vi "Get Connection Count.vi"(8 "error in (no error)":errorcluster, 11 "TCP Socket Server in":refnum<data-value>) -> (0 "error out":errorcluster, 2 "connection count":i32, 3 "TCP Socket Server out":refnum<data-value>)   [LabVIEW 2019, in "TCP Socket Server.lvclass"]
uses:
  TCP Socket Server.lvclass
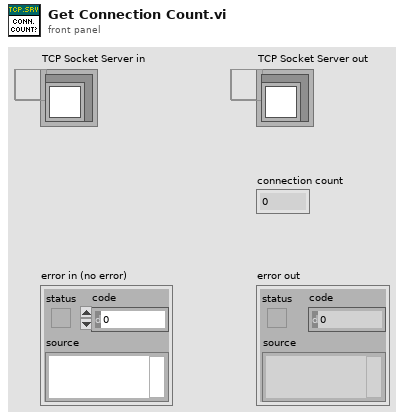
[diagram p1: front panel]
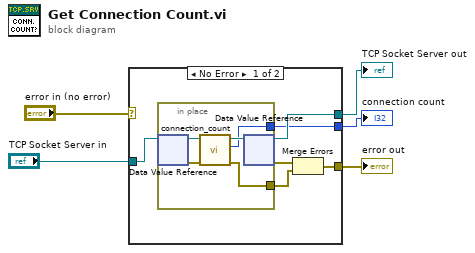
[diagram p0: block diagram]
diagram:
  n1 = case shown="No Error" "error in (no error)" {
    selector: "error in (no error)" -> [_ w18]
    tunnel: [w8 w18] -> w4
    tunnel: [w7 w17] -> w2
    tunnel: "TCP Socket Server in" -> [w11 w17]
    tunnel: [w6 _] -> w1
    frame No Error {
      n2 = in-place {
        in-place-border: [w14] -> w9
        in-place-border: [w12] -> w6
        n3 = in-place-dvr #1(w11) -> (w16:refnum<class "TCP Socket Server.lvclass">, w15:errorcluster)
        n4 = call-dynamic "connection_count.vi"("error in (no error)"=w15, "TCP Socket Server in"=w16) -> ("error out"=w14:errorcluster, "connection count"=w12:i32, "TCP Socket Server out"=w13:refnum<class "TCP Socket Server.lvclass">)  [unwired: 7 in]
        n5 = in-place-dvr #1(w13) -> (w7:refnum<data-value>, w10:errorcluster)
      }
      n6 = Merge Errors(w10, w9) -> (w8:errorcluster)
    }
    frame Error {
    }
  }
  "error out" <- w4
  "TCP Socket Server out" <- w2
  "connection count" <- w1
